vi "Write Register.vi"(8 "error in (no error)":errorcluster, 9 "value":u16, 10 "address":i32, 11 "modbus in":refnum<class "libmodbus.lvclass">) -> (0 "error out":errorcluster, 3 "modbus out":refnum<class "libmodbus.lvclass">)   [LabVIEW 2017, in "libmodbus.lvlib" / "libmodbus.lvclass"]
doc: "Writes single modbus holding register."
uses:
  libmodbus.lvclass
  libmodbus.lvclass/libmodbus.ctl
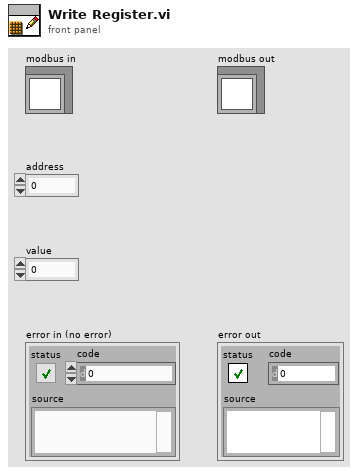
[diagram p1: front panel]
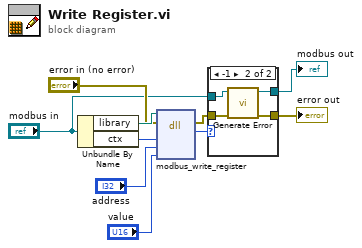
[diagram p0: block diagram]
diagram:
  n1 = Unbundle By Name("modbus in") -> ("library"=w9:path, "ctx"=w10:i64)
  n2 = dll-call lib="?" fn="modbus_write_register"(path in=w9, error in="error in (no error)", "ctx"=w10, "addr"="address", "value"="value") -> (error out=w5:errorcluster, "int"=w7:i32)  [unwired: 4 in, 1 out]
  n3 = case shown="-1" w7 {
    tunnel: [w12 w15] -> w6
    tunnel: w5 -> [w12 w16]
    tunnel: "modbus in" -> [w11 w14]
    tunnel: [w11 w13] -> w3
    frame Default {
    }
    frame -1 {
      n4 = call "Generate Error.vi"("error in (no error)"=w16, "modbus in"=w14) -> ("error out"=w15:errorcluster, "modbus out"=w13:refnum<class "libmodbus.lvclass">)  [unwired: 8 in]
    }
  }
  "modbus out" <- w3
  "error out" <- w6
